vi "serial_write_and_read.vi"(0 "port name in":refnum<visa-resource-name>, 1 "reconnect?":bool, 2 "disconnect?":bool, 3 "timeout (ms)":u32=2000, 5 "write buffer":string, 7 "do writing?":bool, 9 "expecting response?":bool, 11 "error in":errorcluster, 12 "expected max length":u32=255, 13 "connection parameters":T1={"baud rate (9600)"=9600, "data bits (8)"=8, "stop bits (10: 1 bit)"=10, "parity (0:none)"=enum."None", "flow control (0:none)"=0, "timeout (10sec)"=10000, "Enable Termination\nChar (T)"=TRUE, "termination char\n(0xA = '\\n' = LF)\n(0xD = '\\r' = CF) "=13} {"flow control (0:none)" items=["None", "XON/XOFF", "RTS/CTS", "XON/XOFF & RTS/CTS", "DTR/DSR", "XON/XOFF & DTR/DSR"]; "stop bits (10: 1 bit)" items=["1.0"=10, "1.5"=15, "2.0"=20]}, 14 "COM response delay":u32) -> (4 "port name out":refnum<visa-resource-name>, 6 "read buffer":string, 15 "error out":errorcluster)   [LabVIEW 2016]
uses:
  <vilib>/Instr/_visa.llb/VISA Flush IO Buffer Mask.ctl
  <vilib>/Instr/_visa.llb/VISA Set IO Buffer Mask.ctl
  <vilib>/Instr/_visa.llb/VISA Configure Serial Port (Instr).vi
panel:
  out "return count":u32
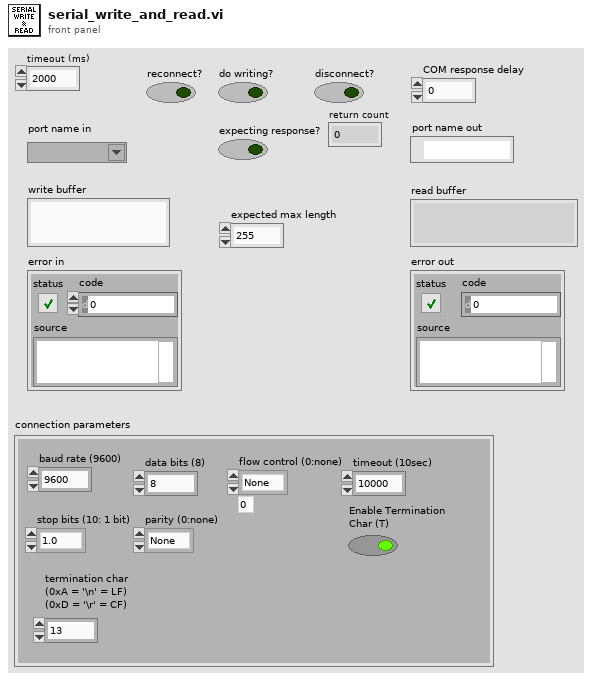
[diagram p1: front panel]
types:
  T1 = cluster{"baud rate (9600)":u32, "data bits (8)":u16, "stop bits (10: 1 bit)":u16, "parity (0:none)":enum16{"None", "Odd", "Even", "Mark", "Space"}, "flow control (0:none)":u16, "timeout (10sec)":u32, "Enable Termination\nChar (T)":bool, "termination char\n(0xA = '\\n' = LF)\n(0xD = '\\r' = CF) ":u8}
  T2 = typedef "VISA Set IO Buffer Mask.ctl" = u16
  T3 = typedef "VISA Flush IO Buffer Mask.ctl" = u16
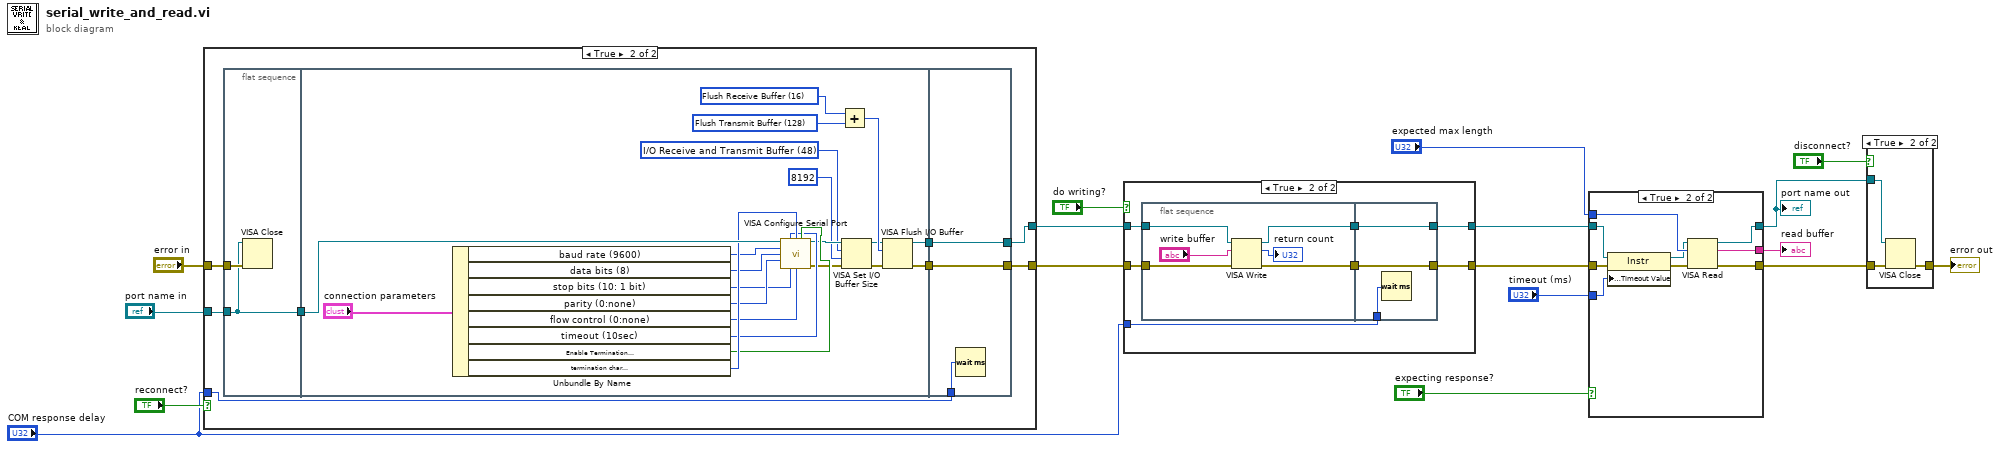
[diagram p0: block diagram]
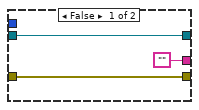
[diagram p5: hidden frame]
diagram:
  n1 = case shown="True" "reconnect?" {
    tunnel: "error in" -> [w18 w26]
    tunnel: [w18 w25] -> w14
    tunnel: [w19 w24] -> w13
    tunnel: "port name in" -> [w19 w23]
    tunnel: "COM response delay" -> [_ w20]
    frame False {
    }
    frame True {
      n2 = flat-sequence {
        tunnel: w26 -> [w29]
        tunnel: [w28] -> w27
        tunnel: w23 -> [w28]
        tunnel: w27 -> [w50]
        tunnel: [w49] -> w22
        tunnel: [w48] -> w21
        tunnel: [w52] -> w24
        tunnel: [w53] -> w25
        tunnel: w22 -> [w53]
        tunnel: w21 -> [w52]
        tunnel: w20 -> [w51]
        frame #0 {
          n3 = VISA Close(VISA resource name=w28, error in (no error)=w29) -> ()  [unwired: 1 out]
        }
        frame #1 {
          w31 = T2 48 items=["I/O Receive Buffer"=16, "I/O Transmit Buffer"=32, "I/O Receive and Transmit Buffer"=48] ("Mask")
          w46 = T3 128 items=["Flush Receive Buffer"=16, "Write Transmit Buffer to Device"=32, "Flush Receive Buffer (No I/O)"=64, "Flush Transmit Buffer"=128] ("Mask")
          w47 = T3 16 items=["Flush Receive Buffer"=16, "Write Transmit Buffer to Device"=32, "Flush Receive Buffer (No I/O)"=64, "Flush Transmit Buffer"=128] ("Mask")
          n4 = Unbundle By Name("connection parameters") -> ("baud rate (9600)"=w36:u32, "data bits (8)"=w37:u16, "stop bits (10: 1 bit)"=w38:u16, "parity (0:none)"=w39:enum16{"None", "Odd", "Even", "Mark", "Space"}, "flow control (0:none)"=w40:u16, "timeout (10sec)"=w41:u32, "Enable Termination\nChar (T)"=w42:bool, "termination char\n(0xA = '\\n' = LF)\n(0xD = '\\r' = CF)"=w43:u8)
          n5 = call-poly "VISA Configure Serial Port"("VISA resource name"=w50, "timeout (10sec)"=w41, "termination char\n(0xA = '\\n' = LF)"=w43, "Enable Termination\nChar (T)"=w42, "baud rate (9600)"=w36, "data bits (8)"=w37, "parity (0:none)"=w39, "stop bits (10: 1 bit)"=w38, "flow control (0:none)"=w40) -> ("VISA resource name out"=w35:refnum<visa-resource-name>, "error out"=w33:errorcluster)  [unwired: 5 in]
          n6 = Add(x=w47, y=w46) -> (x+y=w45:T3)
          n7 = VISA Set I/O Buffer Size(VISA resource name=w35, mask (16)=w31, size (4096)=u32 8192, error in (no error)=w33) -> (VISA resource name out=w34:refnum<visa-resource-name>, error out=w32:errorcluster)
          n8 = VISA Flush I/O Buffer(VISA resource name=w34, mask (16)=w45, error in (no error)=w32) -> (VISA resource name out=w48:refnum<visa-resource-name>, error out=w49:errorcluster)
        }
        frame #2 {
          n9 = Wait (ms)(milliseconds to wait=w51) -> ()  [unwired: 1 out]
        }
      }
    }
  }
  n10 = case shown="True" "do writing?" {
    tunnel: [w54 w62] -> w16
    tunnel: [w55 w61] -> w15
    tunnel: w14 -> [w54 w60]
    tunnel: w13 -> [w55 w59]
    tunnel: "COM response delay" -> [_ w56]
    frame False {
    }
    frame True {
      n11 = flat-sequence {
        tunnel: w60 -> [w66]
        tunnel: w59 -> [w65]
        tunnel: [w68] -> w58
        tunnel: [w67] -> w57
        tunnel: [w70] -> w61
        tunnel: [w71] -> w62
        tunnel: w58 -> [w71]
        tunnel: w57 -> [w70]
        tunnel: w56 -> [w69]
        frame #0 {
          n12 = VISA Write(VISA resource name=w65, write buffer="write buffer", error in (no error)=w66) -> (VISA resource name out=w67:refnum<visa-resource-name>, return count=→"return count":u32, error out=w68:errorcluster)
        }
        frame #1 {
          n13 = Wait (ms)(milliseconds to wait=w69) -> ()  [unwired: 1 out]
        }
      }
    }
  }
  n14 = case shown="True" "expecting response?" {
    tunnel: w16 -> [w73 w76]
    tunnel: w15 -> [w74 w78]
    tunnel: [w73 w83] -> w9
    tunnel: [w74 w82] -> w8
    tunnel: ["" w81] -> w11
    tunnel: "expected max length" -> [_ w80]
    tunnel: "timeout (ms)" -> [_ w79]
    frame False {
    }
    frame True {
      n15 = property class="Instr"(reference=w78, error in=w76, "General Settings:Timeout Value"=w79) -> (reference out=w77:refnum<visa-resource-name>, error out=w75:errorcluster)
      n16 = VISA Read(VISA resource name=w77, byte count=w80, error in (no error)=w75) -> (VISA resource name out=w82:refnum<visa-resource-name>, read buffer=w81:string, error out=w83:errorcluster)  [unwired: 1 out]
    }
  }
  "read buffer" <- w11
  "port name out" <- w8
  n17 = case shown="True" "disconnect?" {
    tunnel: w9 -> [w84 w87]
    tunnel: w8 -> [_ w86]
    tunnel: [w84 w85] -> w3
    frame False {
    }
    frame True {
      n18 = VISA Close(VISA resource name=w86, error in (no error)=w87) -> (error out=w85:errorcluster)
    }
  }
  "error out" <- w3
